vi "CRYDataView SplitterShadow Moving Process.vi"(8 "DataView Index":i32, 9 "Bar_shadow ref":refnum<vi>, 10 "Mouse Pos":T1, 11 "SpliterMoveInfo":T2) -> ()   [LabVIEW 2013]
uses:
  CRYNew View Global.vi
  SubVI/CRYMain Sub Window Global.vi
  <vilib>/Utility/cursorutil.llb/Set Cursor (Icon Pict).vi
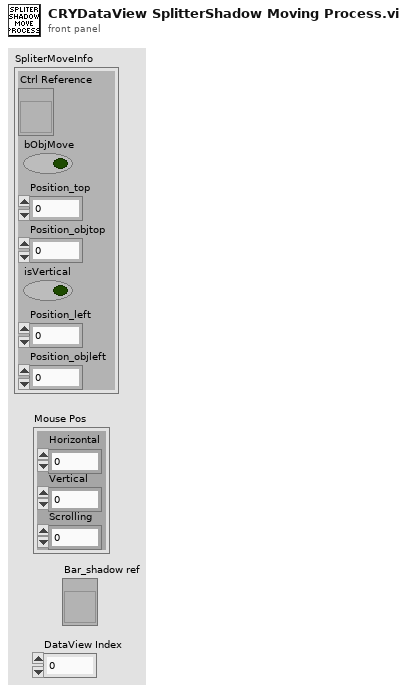
[diagram p1: front panel]
types:
  T1 = cluster{"Horizontal":i32, "Vertical":i32, "Scrolling":i32}
  T2 = cluster{"Ctrl Reference":refnum<vi>, "bObjMove":bool, "Position_top":i32, "Position_objtop":i32, "isVertical":bool, "Position_left":i32, "Position_objleft":i32}
  T3 = typedef "Graph Main Info Cluster.ctl" = cluster{"Selected_BarIdx":i32, "Selected_PanelIdx":i32, "Graph Main VIRef":refnum<vi>, "ToolBarClick":bool, "Spliter Ref Array":refnum<vi>[], "Panel Ref Array":refnum<vi>[], "Spliter_matrix":i32[][], "Panel_matrix":i32[][], "child_spliterIdx_matrix":i32[][], "split_pos_matrix":i32[][], "Title State":bool, "sQueueName":string, "Frame nID":i32, "Graph VIRef Array":cluster{"Graph VIRef":refnum<vi>, "Panel Idx":i32, "Frame VIRef":refnum<vi>, "Icon Ring":i32, "Graph Type":string}[], "View Type":string}
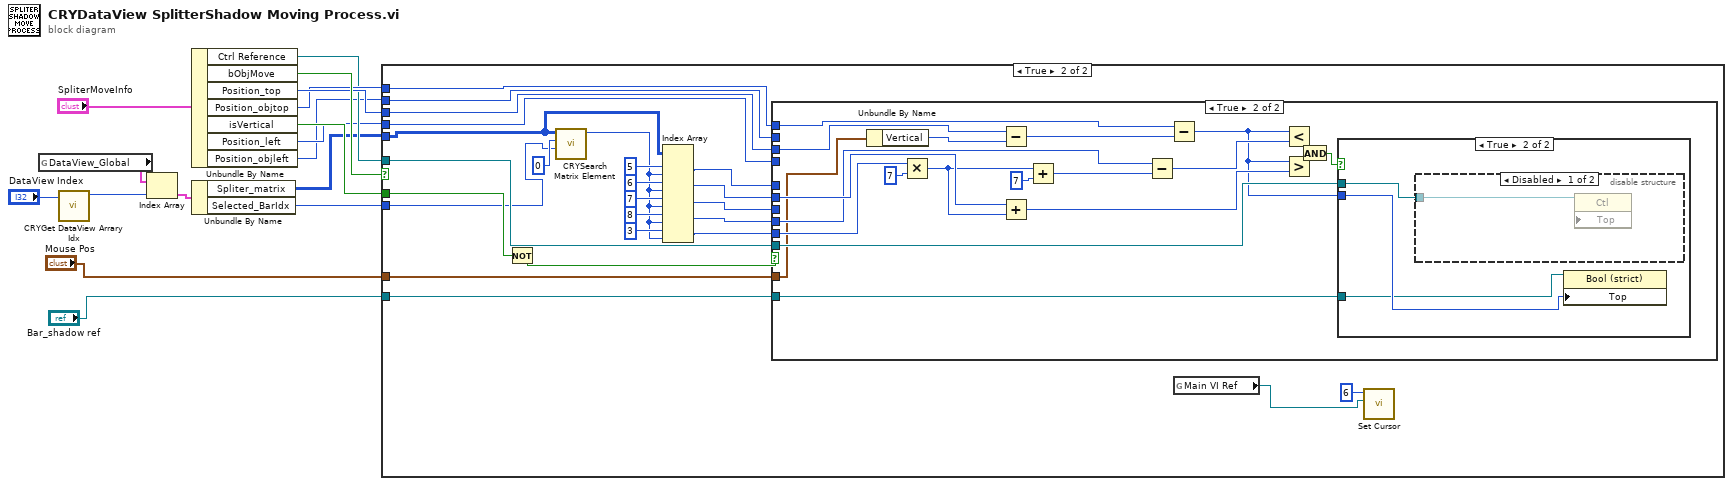
[diagram p0: block diagram]
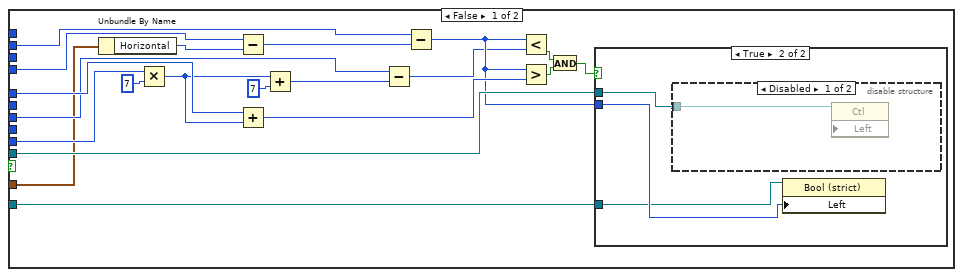
[diagram p3: hidden frame]
diagram:
  n1 = global read "CRYNew View Global.vi" "DataView_Global"() -> (w9:T3[])
  n2 = call "CRYGet DataView Arrary Idx.vi"("DataView Idx In"="DataView Index") -> ("DataView Arrary Idx out"=w1:i32)  [unwired: 10 in]
  n3 = Index Array(array=w9, index=w1) -> (element=w8:T3)
  n4 = Unbundle By Name("SpliterMoveInfo") -> ("Ctrl Reference"=w13:refnum<vi>, "bObjMove"=w16:bool, "Position_top"=w15:i32, "Position_objtop"=w14:i32, "isVertical"=w12:bool, "Position_left"=w11:i32, "Position_objleft"=w10:i32)
  n5 = Unbundle By Name(w8) -> ("Spliter_matrix"=w3:i32[][], "Selected_BarIdx"=w7:i32)
  n6 = case shown="True" w16 {
    tunnel: w13 -> [_ w41]
    tunnel: w15 -> [_ w40]
    tunnel: w14 -> [_ w39]
    tunnel: w12 -> [_ w36]
    tunnel: w11 -> [_ w38]
    tunnel: w10 -> [_ w37]
    tunnel: w3 -> [_ w25]
    tunnel: w7 -> [_ w34]
    tunnel: "Mouse Pos" -> [_ w32]
    tunnel: "Bar_shadow ref" -> [_ w31]
    frame False {
    }
    frame True {
      n7 = Not(x=w36) -> (.not. x?=w33:bool)
      n8 = call "CRYSearch Matrix Element.vi"("element"=w34, "index (row)"=0, "matrix in"=w25) -> ("index of element"=w24:i32)  [unwired: 8 in]
      n9 = Index Array(array=w25, index (row) #1=5 ("index (row)"), index (col) #1=w24, index (row) #2=6 ("index (row)"), index (col) #2=w24, index (row) #3=7 ("index (row)"), index (col) #3=w24, index (row) #4=8 ("index (row)"), index (col) #4=w24, index (row) #5=3 ("index (row)"), index (col) #5=w24) -> (element #1=w23:i32, element #2=w22:i32, element #3=w21:i32, element #4=w20:i32, element #5=w19:i32)
      n10 = case shown="True" w33 {
        tunnel: w41 -> [w59 w85]
        tunnel: w40 -> [_ w84]
        tunnel: w39 -> [_ w83]
        tunnel: w38 -> [w58 _]
        tunnel: w37 -> [w57 _]
        tunnel: w23 -> [w56 _]
        tunnel: w21 -> [w52 _]
        tunnel: w22 -> [_ w80]
        tunnel: w20 -> [_ w78]
        tunnel: w19 -> [w48 w72]
        tunnel: w32 -> [w43 w67]
        tunnel: w31 -> [w42 w66]
        frame False {
          n11 = Unbundle By Name(w43) -> ("Horizontal"=w60:i32)
          n12 = Multiply(x=w48, y=7) -> (x*y=w45:i32)
          n13 = Subtract(x=w58, y=w60) -> (x-y=w61:i32)
          n14 = Add(x=w56, y=w45) -> (x+y=w55:i32)
          n15 = Add(x=w45, y=7) -> (x+y=w44:i32)
          n16 = Subtract(x=w52, y=w44) -> (x-y=w53:i32)
          n17 = Subtract(x=w57, y=w61) -> (x-y=w54:i32)
          n18 = Less?(x=w54, y=w53) -> (x < y?=w51:bool)
          n19 = Greater?(x=w54, y=w55) -> (0:w50:bool)
          n20 = And(x=w51, y=w50) -> (x .and. y?=w49:bool)
          n21 = case shown="True" w49 {
            tunnel: w59 -> [_ w64]
            tunnel: w54 -> [_ w63]
            tunnel: w42 -> [_ w62]
            frame False {
            }
            frame True {
              n22 = disable-structure shown="Disabled" {
                disable-tunnel: w64 -> [w65 _]
                frame Disabled {
                  n23 = property class="Ctl" props=["Left"](reference=w65) -> ()  [unwired: 2 in, 2 out]
                }
                frame Enabled {
                }
              }
              n24 = property class="Bool (strict)"(reference=w62, "Left"=w63) -> ()  [unwired: 1 in, 2 out]
            }
          }
        }
        frame True {
          n25 = Unbundle By Name(w67) -> ("Vertical"=w81:i32)
          n26 = Multiply(x=w72, y=7) -> (x*y=w70:i32)
          n27 = Subtract(x=w84, y=w81) -> (x-y=w82:i32)
          n28 = Add(x=w80, y=w70) -> (x+y=w79:i32)
          n29 = Add(x=w70, y=7) -> (x+y=w68:i32)
          n30 = Subtract(x=w78, y=w68) -> (x-y=w77:i32)
          n31 = Subtract(x=w83, y=w82) -> (x-y=w76:i32)
          n32 = Less?(x=w76, y=w77) -> (x < y?=w75:bool)
          n33 = Greater?(x=w76, y=w79) -> (0:w74:bool)
          n34 = And(x=w75, y=w74) -> (x .and. y?=w73:bool)
          n35 = case shown="True" w73 {
            tunnel: w85 -> [_ w88]
            tunnel: w76 -> [_ w87]
            tunnel: w66 -> [_ w86]
            frame False {
            }
            frame True {
              n36 = disable-structure shown="Disabled" {
                disable-tunnel: w88 -> [w89 _]
                frame Disabled {
                  n37 = property class="Ctl" props=["Top"](reference=w89) -> ()  [unwired: 2 in, 2 out]
                }
                frame Enabled {
                }
              }
              n38 = property class="Bool (strict)"(reference=w86, "Top"=w87) -> ()  [unwired: 1 in, 2 out]
            }
          }
        }
      }
      n39 = global read "CRYMain Sub Window Global.vi" "Main VI Ref"() -> (w17:refnum<vi>)
      n40 = call-poly <vilib>:"Set Cursor.vi"("VI reference (current VI)"=w17, "icon"=u16 6) -> ()  [unwired: 1 in, 9 out]
    }
  }
